vi "AudioStreamer.Set Num Reps.vi"(0 "nreps":i32, 11 "error in (no error)":errorcluster) -> (15 "error out":errorcluster)   [LabVIEW 2020]
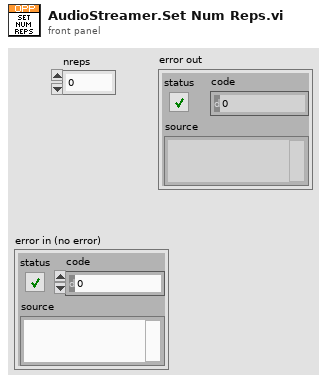
[diagram p1: front panel]
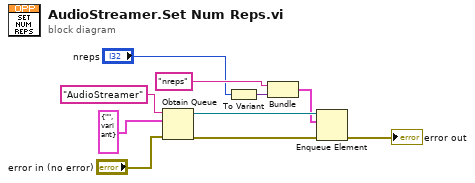
[diagram p0: block diagram]
diagram:
  n1 = Obtain Queue(name (unnamed)="AudioStreamer", element data type=cluster{string, variant} {"", variant}, error in (no error)="error in (no error)") -> (queue out=w7:refnum<queue>, error out=w8:errorcluster)  [unwired: 2 in, 1 out]
  n2 = To Variant(anything="nreps") -> (Variant=w5:variant)
  n3 = Bundle("nreps", "Variant"=w5) -> (w3:cluster{string, "Variant":variant})  [unwired: 1 in]
  n4 = Enqueue Element(queue=w7, element=w3, error in (no error)=w8) -> (error out=→"error out":errorcluster)  [unwired: 1 in, 2 out]
